vi "XImc simple example.vi"() -> ()   [LabVIEW 2012]
uses:
  libximc.lvlib
panel:
  in  "error in (no error)":errorcluster
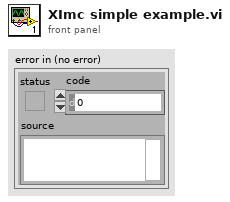
[diagram p1: front panel]
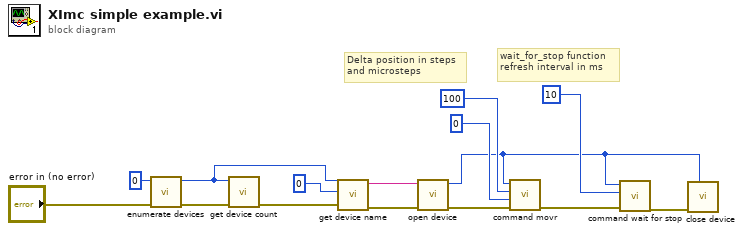
[diagram p0: block diagram]
diagram:
  # "Delta position in steps and microsteps"
  # "wait_for_stop function refresh interval in ms"
  n1 = call "enumerate devices.vi"("error in (no error)"="error in (no error)", "enumerate_flags"=0 ("probe_devices")) -> ("error out"=w13:errorcluster, "function return"=w11:u64)  [unwired: 8 in]
  n2 = call "get device count.vi"("error in (no error)"=w13, "device_enumeration"=w11) -> ("error out"=w12:errorcluster)  [unwired: 8 in, 1 out]
  n3 = call "get device name.vi"("error in (no error)"=w12, "device_index"=0 ("probe_devices"), "device_enumeration"=w11) -> ("error out"=w8:errorcluster, "function return"=w9:string)  [unwired: 7 in]
  n4 = call "open device.vi"("error in (no error)"=w8, "name"=w9) -> ("error out"=w6:errorcluster, "function return"=w1:i32)  [unwired: 8 in]
  n5 = call "command movr.vi"("error in (no error)"=w6, "uDeltaPosition"=0 ("probe_devices"), "DeltaPosition"=100 ("probe_devices"), "id"=w1) -> ("error out"=w5:errorcluster)  [unwired: 6 in, 1 out]
  n6 = call "command wait for stop.vi"("error in (no error)"=w5, "refresh_interval_ms"=10 ("probe_devices"), "id"=w1) -> ("error out"=w3:errorcluster)  [unwired: 7 in, 1 out]
  n7 = call "close device.vi"("error in (no error)"=w3, "id"=w1) -> ()  [unwired: 7 in, 3 out]
